vi "MT Calculate BER.vi"   [LabVIEW 2020, in "niDMT.lvlib"]
doc: "Calculates the average bit error rate (BER) against a PN sequence or a reference bit pattern that you specify."
uses:
  <vilib>/addons/Modulation/niDMT.lvlib
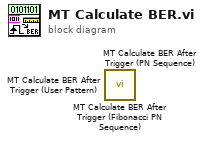
[diagram p0: block diagram]
diagram:
  n1 = call <vilib>:"MT Calculate BER After Trigger (Fibonacci PN Sequence).vi"() -> ()  [unwired: 11 in, 5 out]
  n2 = call <vilib>:"MT Calculate BER After Trigger (PN Sequence).vi"() -> ()  [unwired: 11 in, 5 out]
  n3 = call <vilib>:"MT Calculate BER After Trigger (User Pattern).vi"() -> ()  [unwired: 11 in, 5 out]
